vi "test1.vi"() -> ()   [LabVIEW 2019]
uses:
  <vilib>/vision/Image Controls.llb/IMAQ Image.ctl
  <resource>/objmgr/IMAQImage.rc
  EmergentCameraC/EmergentCameraC.lvlib
panel:
  in  "New Image":T1
  in  "stop":bool
  out "Transfer Max Size":i32
  out "LineWidth(Pixels)":i32
  out "Image":T1(plugin-control)
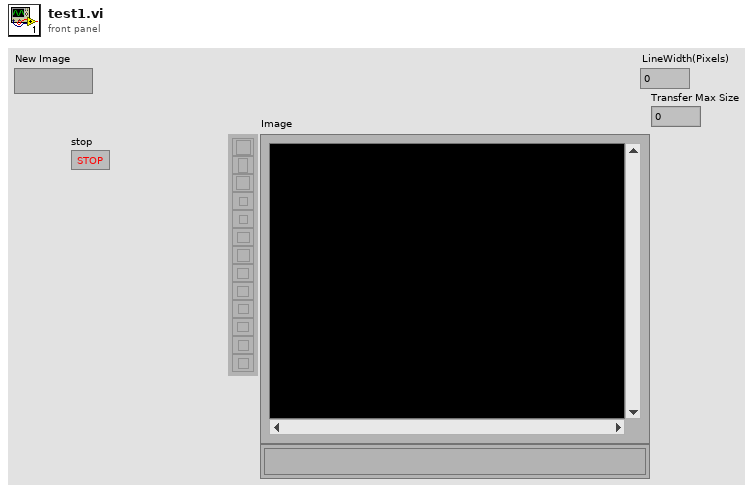
[diagram p1: front panel]
types:
  T1 = typedef "IMAQ Image.ctl" = refnum<image>
  T2 = typedef "Image Type" = u32
  T3 = enum32{"Map Pixel Pointer", "Unmap Pixel Pointer", "Get Pixels Infos"}
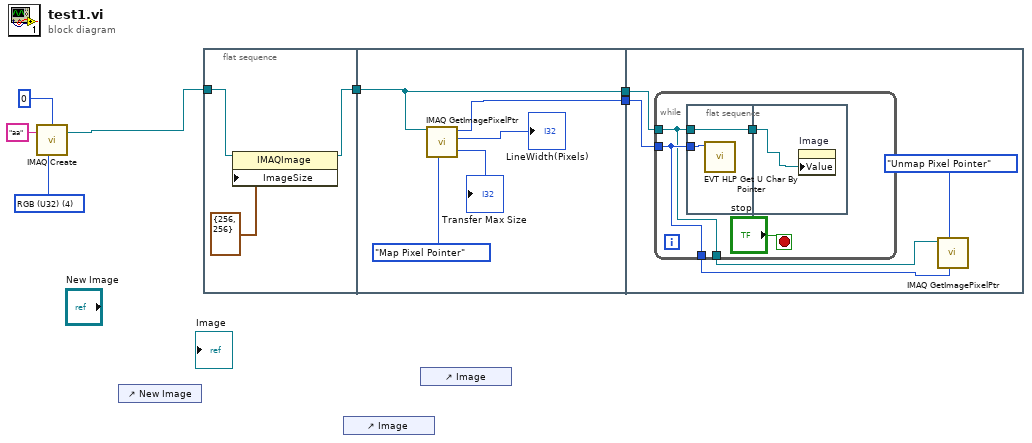
[diagram p0: block diagram]
diagram:
  w5 = T2 4 items=["Grayscale (U8)", "Grayscale (I16)", "Grayscale (SGL)", "Complex (CSG)", "RGB (U32)", "HSL (U32)", "RGB (U64)", "Grayscale (U16)"] ("Image Type")
  n1 = call "IMAQ Create"("Border Size"=0, "Image Name"="aa", "Image Type"=w5) -> ("New Image"=w7:T1)  [unwired: 2 in, 1 out]
  n2 = control-ref of="New Image"() -> ()  [unwired: 1 out]
  n3 = flat-sequence {
    tunnel: w7 -> [w10]
    tunnel: [w9] -> w4
    tunnel: w4 -> [w14]
    tunnel: [w14] -> w2
    tunnel: [w11] -> w1
    tunnel: w2 -> [w19]
    tunnel: w1 -> [w20]
    frame #0 {
      n4 = property class="IMAQImage"(reference=w10, "ImageSize"=cluster{"x":i32, "y":i32} {"x"=256, "y"=256} ("Image Size")) -> (reference out=w9:T1)  [unwired: 1 in, 1 out]
    }
    frame #1 {
      n5 = call "IMAQ GetImagePixelPtr"("Function"=T3."Map Pixel Pointer", "Image"=w14) -> ("LineWidth(Pixels)"=→"LineWidth(Pixels)":i32, "Pixel Pointer out"=w11:u64, "Transfer Max Size"=→"Transfer Max Size":i32)  [unwired: 4 in, 3 out]
    }
    frame #2 {
      n6 = while {
        tunnel: w20 -> [w22]
        tunnel: w19 -> [w21]
        tunnel: [w22] -> w18
        tunnel: [w21] -> w16
        stop <- "stop" stop-if-true
        n7 = flat-sequence {
          tunnel: w22 -> [w26]
          tunnel: [w25] -> w23
          tunnel: w21 -> [w25]
          tunnel: w23 -> [w27]
          frame #0 {
            n8 = call "EVT HLP Get U Char By Pointer.vi"("ptr"=w26) -> ()  [unwired: 10 in, 1 out]
          }
          frame #1 {
            n9 = property on="Image" class="ImageControl"("Value"=w27) -> ()  [unwired: 2 in, 2 out]
          }
        }
      }
      n10 = call "IMAQ GetImagePixelPtr"("Pixel Pointer in"=w18, "Function"=T3."Unmap Pixel Pointer", "Image"=w16) -> ()  [unwired: 3 in, 6 out]
    }
  }
  n11 = control-ref of="Image"() -> ()  [unwired: 1 out]
  n12 = control-ref of="Image"() -> ()  [unwired: 1 out]
